vi "Init.vi"(8 "error in":errorcluster, 10 "Section Name":string, 11 "Section Name in":refnum<class "Section Name.lvclass">) -> (0 "error out":errorcluster, 3 "Section Name out":refnum<class "Section Name.lvclass">)   [LabVIEW 2019, in "Electronic Datasheet.lvlib" / "Section Name.lvclass"]
uses:
  Section Name.lvclass
  Section Name.lvclass/Section Name.ctl
  Electronic Datasheet.lvlib
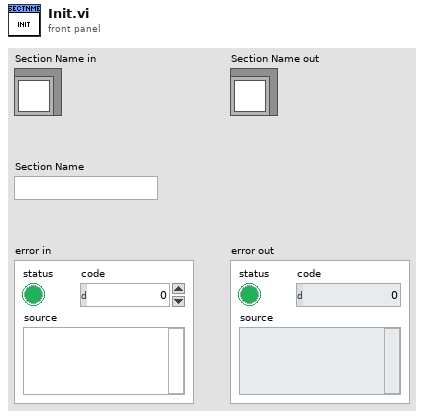
[diagram p1: front panel]
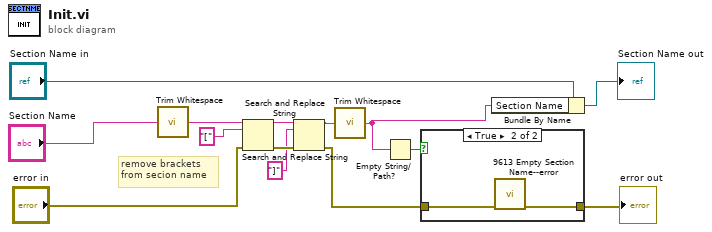
[diagram p0: block diagram]
diagram:
  # "remove brackets\nfrom secion name"
  n1 = call <vilib>:"Trim Whitespace.vi"("string"="Section Name") -> ("trimmed string"=w11:string)  [unwired: 1 in]
  n2 = Search and Replace String(input string=w11, search string="[" ("search string/char (-)"), error in="error in") -> (result string=w9:string, error out=w8:errorcluster)  [unwired: 5 in, 2 out]
  n3 = Search and Replace String(input string=w9, search string="]" ("search string/char (-)"), error in=w8) -> (result string=w5:string, error out=w6:errorcluster)  [unwired: 5 in, 2 out]
  n4 = call <vilib>:"Trim Whitespace.vi"("string"=w5) -> ("trimmed string"=w2:string)  [unwired: 1 in]
  n5 = Empty String/Path?(string/path=w2) -> (empty?=w12:bool)
  n6 = case shown="True" w12 {
    tunnel: w6 -> [w15 w17]
    tunnel: [w15 w16] -> w3
    frame False {
    }
    frame True {
      n7 = call "9613 Empty Section Name--error.vi"("error in"=w17) -> ("error out"=w16:errorcluster)  [unwired: 10 in]
    }
  }
  "error out" <- w3
  n8 = Bundle By Name(cluster="Section Name in", "Section Name"=w2) -> (→"Section Name out":refnum<class "Section Name.lvclass">)
